vi "Write Wavenames.vi"(8 "error in (no error)":errorcluster, 10 "Wavenames":string[](array[string]), 11 "LVtoITX in":refnum<class "LVtoITX.lvclass">) -> (0 "error out":errorcluster, 3 "LVtoITX out":refnum<class "LVtoITX.lvclass">)   [LabVIEW 2016, in "LVtoITX.lvclass"]
uses:
  LVtoITX.lvclass
  LVtoITX.lvclass/LVtoITX.ctl
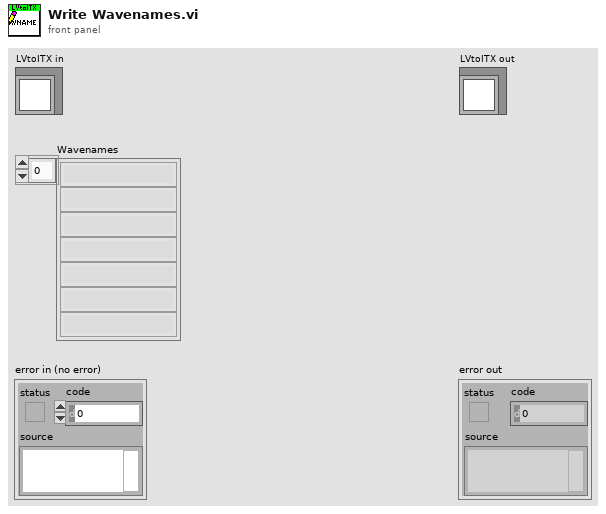
[diagram p1: front panel]
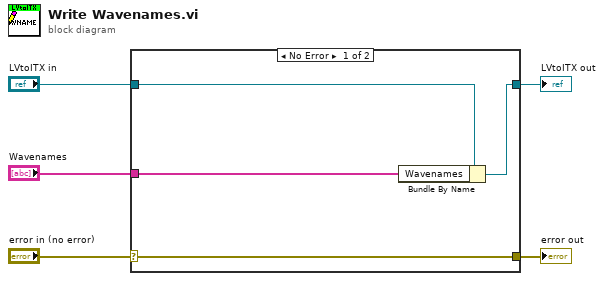
[diagram p0: block diagram]
diagram:
  n1 = case shown="No Error" "error in (no error)" {
    selector: "error in (no error)" -> [w9 w10]
    tunnel: [w9 w10] -> w4
    tunnel: [w7 w11] -> w2
    tunnel: "LVtoITX in" -> [w8 w11]
    tunnel: "Wavenames" -> [w6 _]
    frame No Error {
      n2 = Bundle By Name(cluster=w8, "Wavenames"=w6) -> (w7:refnum<class "LVtoITX.lvclass">)
    }
    frame Error {
    }
  }
  "error out" <- w4
  "LVtoITX out" <- w2
